vi "CRYCheck Sub Data View.vi"(10 "VI Refnum":refnum<vi>, 11 "Window Name":string) -> (3 "data view?":bool)   [LabVIEW 2013]
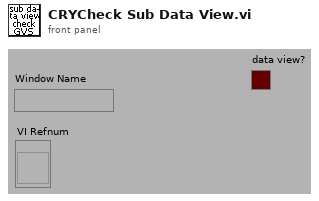
[diagram p1: front panel]
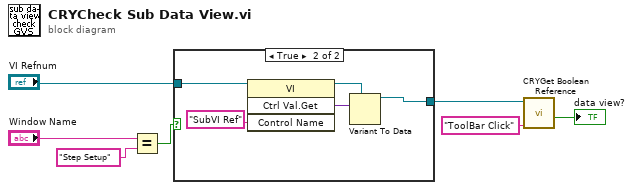
[diagram p0: block diagram]
diagram:
  n1 = Equal?(x="Window Name", y="Step Setup" ("Window Name")) -> (x = y?=w4:bool)
  n2 = case shown="True" w4 {
    tunnel: "VI Refnum" -> [w8 w13]
    tunnel: [w8 w9] -> w3
    frame False {
    }
    frame True {
      n3 = invoke class="VI" method="Ctrl Val.Get"(reference=w13, "Control Name"="SubVI Ref" ("Label Name")) -> (reference out=w10:refnum<vi>, "Get Control Value Variant"=w11:variant)  [unwired: 2 in, 2 out]
      n4 = Variant To Data(type=w10, Variant=w11) -> (data=w9:refnum<vi>)  [unwired: 1 in, 1 out]
    }
  }
  n5 = call "CRYGet Boolean Reference.vi"("Label Name"="ToolBar Click", "VI Refnum"=w3) -> ("Exist?"=→"data view?":bool)  [unwired: 9 out]
